vi "Yield (async) JSON.vi"(4 "ArgumentsKw":string, 6 "Arguments":string, 7 "Options":string, 8 "error in (no error)":errorcluster, 10 "Invocation Request":refnum<class "Invocation Request ID.lvclass">, 11 "WAMP Client in":refnum<class "WAMP Client.lvclass">) -> (0 "error out":errorcluster, 3 "WAMP Client out":refnum<class "WAMP Client.lvclass">)   [LabVIEW 2020, in "wamplv.lvlib" / "WAMP Client.lvclass"]
uses:
  WAMP Client.lvclass
  WAMP Client.lvclass/WAMP Client.ctl
  Private/Requests/Yield/Yield JSON/Yield JSON.lvclass
  C:/local/wamplv/Private/Requests/Yield/IYield/IYield.lvclass
  C:/local/wamplv/Private/Requests/IGenericWithOutputInternalMessage/IGenericWithOutputInternalMessage/IGenericWithOutputInternalMessage.lvclass
  C:/local/wamplv/Private/Requests/IInternalMessage/IInternalMessage.lvclass
  C:/local/wamplv/Private/Requests/Yield/Yield JSON/Yield JSON.lvclass
  Private/Invocation Request ID/Invocation Request ID.lvclass
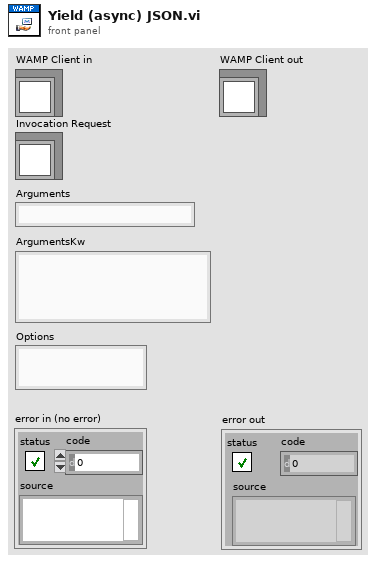
[diagram p1: front panel]
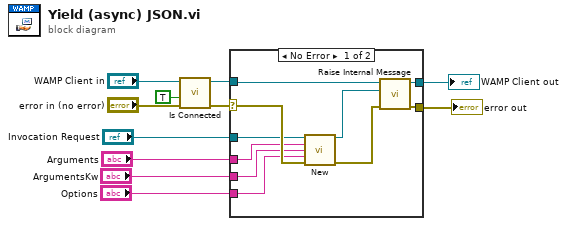
[diagram p0: block diagram]
diagram:
  n1 = call "Is Connected.vi"("error in"="error in (no error)", "Raise error if not connected"=TRUE, "WAMP Client in"="WAMP Client in") -> ("error out"=w4:errorcluster, "WAMP Client out"=w5:refnum<class "WAMP Client.lvclass">)  [unwired: 6 in, 1 out]
  n2 = case shown="No Error" w4 {
    selector: w4 -> [w18 w23]
    tunnel: [w19 w23] -> w11
    tunnel: [w20 w22] -> w10
    tunnel: w5 -> [w21 w22]
    tunnel: "ArgumentsKw" -> [w15 _]
    tunnel: "Arguments" -> [w16 _]
    tunnel: "Options" -> [w14 _]
    tunnel: "Invocation Request" -> [w17 _]
    frame No Error {
      n3 = call "New.vi"("Invocation Request"=w17, "Arguments"=w16, "ArgumentsKw"=w15, "Options"=w14, "error in (no error)"=w18) -> ("Yield JSON out"=w13:refnum<class "Yield JSON.lvclass">, "error out"=w12:errorcluster)  [unwired: 9 in]
      n4 = call "Raise Internal Message.vi"("error in (no error)"=w12, "IInternalMessage"=w13, "WAMP Client in"=w21) -> ("error out"=w19:errorcluster, "WAMP Client out"=w20:refnum<class "WAMP Client.lvclass">)  [unwired: 7 in]
    }
    frame Error {
    }
  }
  "error out" <- w11
  "WAMP Client out" <- w10
